vi "Query Output.vi"(8 "error in":errorcluster, 11 "SL_SC in":refnum<class "SL_SC.lvclass">) -> (0 "error out":errorcluster, 1 "Output":u8[](array[numeric]), 3 "SL_SC out":refnum<class "SL_SC.lvclass">)   [LabVIEW 2019, in "SL_SC.lvlib" / "SL_SC.lvclass"]
doc: "This method must be overridden by the child class.\n\nThis should read the status at the output of the device and return a weform capture of the named signal states."
uses:
  Library/SL_SC.lvclass
  Library/SL_SC.lvclass/SL_SC.ctl
  <vilib>/SLSC/Get Generic Property (U32).vi
  <vilib>/SLSC/SLSC.lvlib
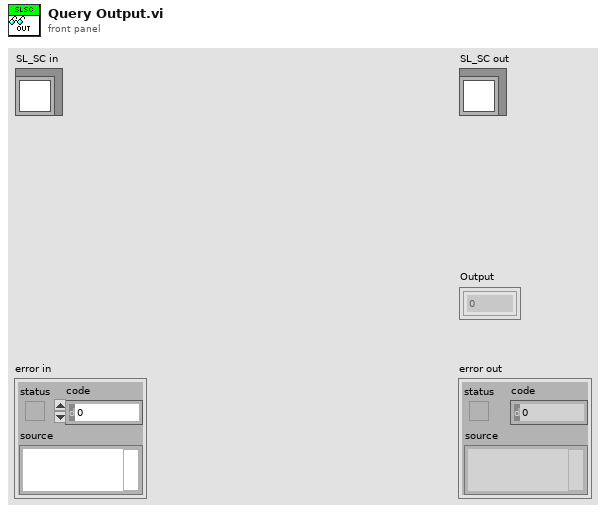
[diagram p1: front panel]
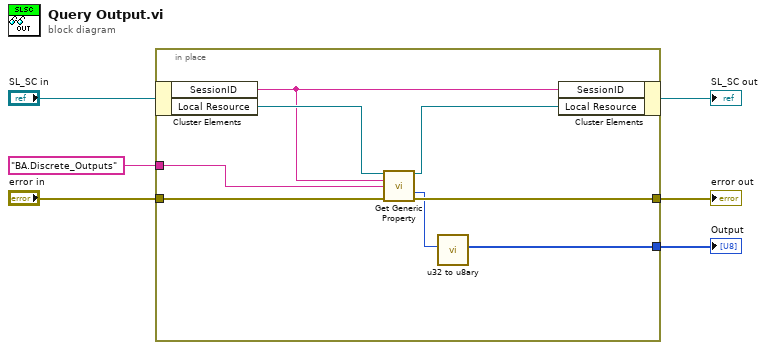
[diagram p0: block diagram]
diagram:
  n1 = in-place {
    in-place-border: [w14] -> w4
    in-place-border: "error in" -> [w13]
    in-place-border: [w12] -> w2
    in-place-border: "BA.Discrete_Outputs" -> [w11]
    n2 = in-place-cluster #1("SL_SC in") -> ("SessionID"=w7:string, "Local Resource"=w9:refnum<k21>)
    n3 = call-poly <vilib>:"Get Generic Property.vi"("session in"=w9, "resources"=w7, "property"=w11, "error in (no error)"=w13) -> ("session out"=w8:refnum<k21>, "property value"=w10:u32, "error out"=w12:errorcluster)  [unwired: 9 in]
    n4 = call "u32 to u8ary.vi"("Numeric"=w10) -> ("Array"=w14:u8[])  [unwired: 10 in]
    n5 = in-place-cluster #1("SessionID"=w7, "Local Resource"=w8) -> (→"SL_SC out":refnum<class "SL_SC.lvclass">)
  }
  "error out" <- w2
  "Output" <- w4
